vi "Get All Symbol Information.vi"(8 "error in (no error)":errorcluster, 11 "TwinCAT ADS in":refnum<class "TwinCAT ADS.lvclass">) -> (0 "error out":errorcluster, 1 "Symbol Collection":refnum<k24>, 3 "TwinCAT ADS out":refnum<class "TwinCAT ADS.lvclass">)   [LabVIEW 2018, in "TwinCAT ADS.lvclass"]
uses:
  TwinCAT ADS.lvclass
  TwinCAT.Ads
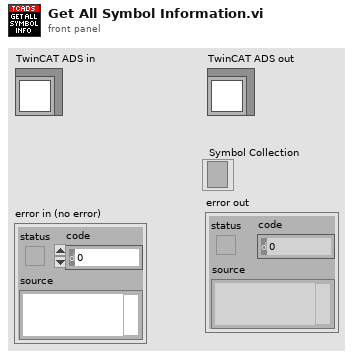
[diagram p1: front panel]
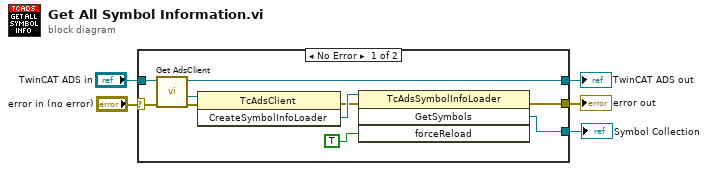
[diagram p0: block diagram]
diagram:
  n1 = case shown="No Error" "error in (no error)" {
    selector: "error in (no error)" -> [w10 w17]
    tunnel: [w8 w17] -> w4
    tunnel: [w7 w16] -> w2
    tunnel: "TwinCAT ADS in" -> [w9 w16]
    tunnel: [w6 _] -> w1
    frame No Error {
      n2 = call-dynamic "Get AdsClient.vi"("error in (no error)"=w10, "TwinCAT ADS in"=w9) -> ("error out"=w12:errorcluster, ".NET TcAdsClient refnum"=w11:refnum<k24>, "TwinCAT ADS out"=w7:refnum<class "TwinCAT ADS.lvclass">)  [unwired: 7 in]
      n3 = invoke class="TcAdsClient" method="CreateSymbolInfoLoader"(reference=w11, error in=w12) -> (error out=w14:errorcluster, "CreateSymbolInfoLoader"=w15:refnum<k24>)  [unwired: 1 in, 1 out]
      n4 = invoke class="TcAdsSymbolInfoLoader" method="GetSymbols"(reference=w15, error in=w14, "forceReload"=TRUE) -> (error out=w8:errorcluster, "GetSymbols"=w6:refnum<k24>)  [unwired: 1 in, 2 out]
    }
    frame Error {
    }
  }
  "error out" <- w4
  "TwinCAT ADS out" <- w2
  "Symbol Collection" <- w1
